vi "Close Client.vi"(8 "error in":errorcluster, 11 "ClientID in":T1) -> (0 "error out":errorcluster)   [LabVIEW 2019, in "grpc-lvsupport.lvlib"]
uses:
  grpc-lvsupport.lvlib
  grpcId.ctl
  <vilib>/Utility/error.llb/Error Cluster From Error Code.vi
  <resource>/labview_grpc_server.dll
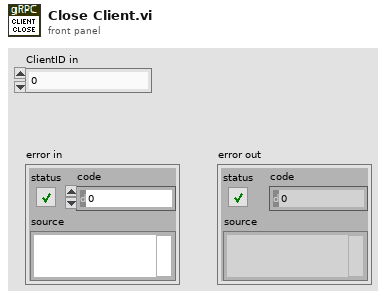
[diagram p1: front panel]
types:
  T1 = typedef "grpc-lvsupport.lvlib/grpcId.ctl" = u64
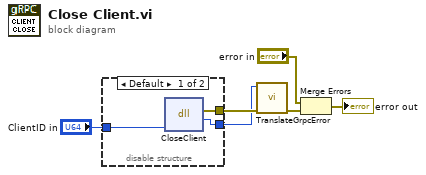
[diagram p0: block diagram]
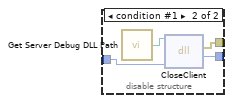
[diagram p2: hidden frame]
diagram:
  n1 = disable-structure shown="Default" {
    disable-tunnel: [w9 w13] -> w6
    disable-tunnel: "ClientID in" -> [w8 w11]
    disable-tunnel: [w7 w10] -> w4
    frame condition #0 (active) {
      n2 = dll-call lib="C:/Program Files (x86)/National Instruments/LabVIEW 2024/resource/labview_grpc_server.*" fn="CloseClient"("clientId"=w8) -> (error out=w9:errorcluster, "return type"=w7:i32)  [unwired: 4 in, 1 out]
    }
    frame condition #1 {
      n3 = call "Get Server Debug DLL Path.vi"() -> ("DLL Path"=w12:path)
      n4 = dll-call lib="?" fn="CloseClient"(path in=w12, "clientId"=w11) -> (error out=w13:errorcluster, "return type"=w10:i32)  [unwired: 3 in, 1 out]
    }
  }
  n5 = call "TranslateGrpcError.vi"("error in"=w6, "Error Code"=w4) -> ("error out"=w2:errorcluster)  [unwired: 9 in]
  n6 = Merge Errors("error in", w2) -> (→"error out":errorcluster)
